vi "set name.vi"(8 "error in (no error)":errorcluster caption="에러 입력(에러 없음)", 11 "Auto Track Wave 입력":refnum<class "Auto Track Wave.lvclass">) -> (0 "error out":errorcluster caption="에러 출력", 3 "Auto Track Wave 출력":refnum<class "Auto Track Wave.lvclass">)   [LabVIEW 2020, in "Auto Track Wave.lvclass"]
uses:
  Auto Track Wave.lvclass
  Waveform Gen/Waveform Gen.lvclass/Waveform Gen.ctl
  Waveform Obj/Waveform Obj.lvclass/Waveform Obj.ctl
  Waveform Gen/Accessors/Read frequency.vi
  Waveform Obj/Accessors/Write name.vi
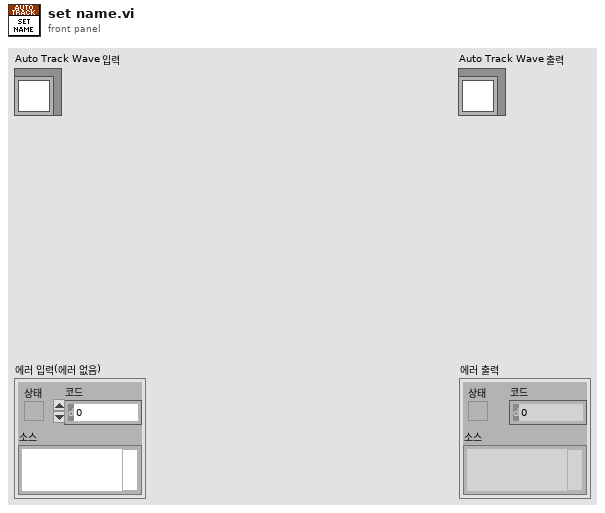
[diagram p1: front panel]
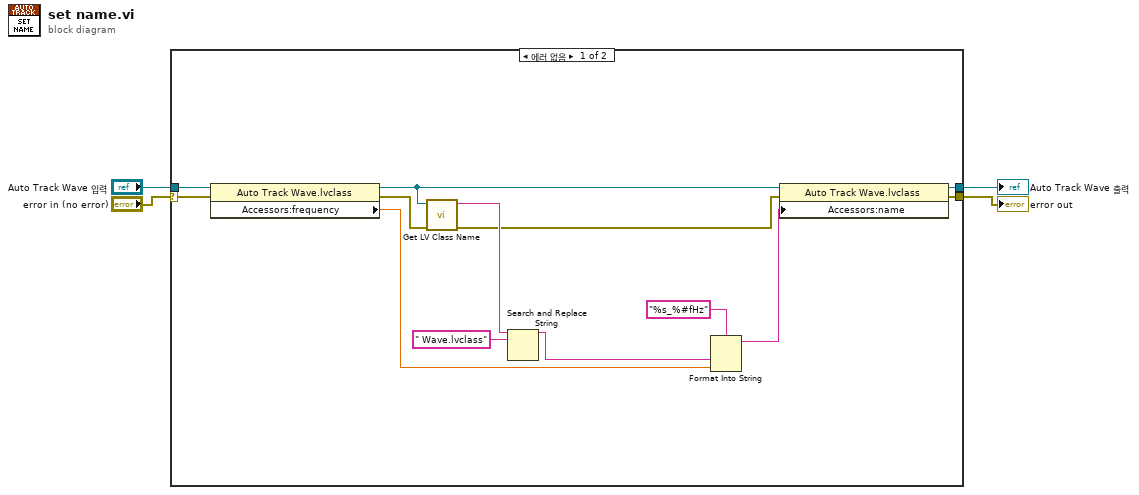
[diagram p0: block diagram]
diagram:
  n1 = case shown="에러 없음" "error in (no error)" {
    selector: "error in (no error)" -> [w15 w18]
    tunnel: "Auto Track Wave 입력" -> [w14 w19]
    tunnel: [w12 w18] -> w4
    tunnel: [w11 w19] -> w3
    frame No Error {
      n2 = property class="Auto Track Wave.lvclass"(reference=w14, error in=w15) -> (reference out=w10:refnum<class "Auto Track Wave.lvclass">, error out=w13:errorcluster, "Accessors:frequency"=w16:dbl)
      n3 = call <vilib>:"Get LV Class Name.vi"("error in (no error)"=w13, "object"=w10) -> ("error out"=w8:errorcluster, "class name"=w9:string)  [unwired: 8 in]
      n4 = Search and Replace String(input string=w9, search string=" Wave.lvclass" ("검색 문자열")) -> (result string=w5:string)  [unwired: 6 in, 3 out]
      n5 = Format Into String(format string="%s_%#fHz" ("포맷 문자열"), w5, w16) -> (resulting string=w7:string)  [unwired: 2 in, 1 out]
      n6 = property class="Auto Track Wave.lvclass"(reference=w10, error in=w8, "Accessors:name"=w7) -> (reference out=w11:refnum<class "Auto Track Wave.lvclass">, error out=w12:errorcluster)
    }
    frame Error {
    }
  }
  "error out" <- w4
  "Auto Track Wave 출력" <- w3
